vi "Manual Roller Control.vi"() -> (1 "Boolean":bool, 2 "Right Speed Out":dbl, 3 "Left Speed Out":dbl)   [LabVIEW 2014]
uses:
  Really Real Manual Align.ctl
  Robot Global Data.vi
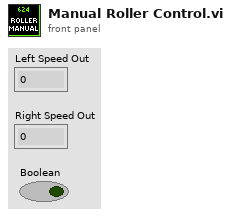
[diagram p1: front panel]
types:
  T1 = typedef "Really Real Manual Align.ctl" = enum16{"In", "Left", "Right", "Out", "Idle", "HP Load", "Speeds"}
  T2 = typedef "Dashboard Control Data.ctl" = cluster{"Cam Exposure":dbl, "Go to angle":dbl, "Steer PID Gains":cluster{"proportional gain (Kc)":dbl, "integral time (Ti, min)":dbl, "derivative time (Td, min)":dbl}, "Steer PID output Range":cluster{"output high":dbl, "output low":dbl}, "Pressure m \nValue":dbl, "Pressure b \nValue":dbl, "Roller Command Cluster ":T3, "Elevator":T4, "Encoder Control":T6, "Auton Settings":cluster{"Drive Dist Window Size":dbl}, "Drivetrain Settings":T7, "Lance":T8}
  T3 = typedef "Roller Control.ctl" = cluster{"Intake Speed":dbl, "Turn In Speed":dbl, "Unload Speed":dbl, "Turn Out Speed":dbl, "Ping Align Tolerance":dbl, "Tote Range Threshold":dbl, "Right Pot 0":dbl, "Pot Threshold":dbl, "Left Pot 0":dbl, "Manual 0s?":bool, "Right Pot Scale":dbl, "Left Pot Scale":dbl, "0 wait time":i32, "Zero Pots":bool, "Min Elevator Height":dbl, "Eject Time":dbl, "Eject US Threshold":dbl, "Anti-Twitch Time":u32, "Ping Caring Threshold":dbl, "Pot Diff Threshold":dbl, "Pinch Sustain":u32, "Absorb Give Up Threshold":dbl, "Untip In Threshold":dbl, "Untip Grab Range":dbl, "Ultrasonic Hold Time":u32, "Landscape Absorb Time":u32, "Pot Use Wait Time":u32, "Can Turn Stop Range":dbl, "Ignore Pressure":bool, "HP Load Speed":dbl}
  T4 = typedef "Elevator DB Control.ctl" = cluster{"PID Output Range":cluster{"output high":dbl, "output low":dbl}, "PID gains":cluster{"proportional gain (Kc)":dbl, "integral time (Ti, min)":dbl, "derivative time (Td, min)":dbl}, "Height Tolerance":sgl, " Encoder Constant":dbl, "Safe Mode Max Speed":sgl, "Eject Time":sgl, "Zeroing Speed":sgl, "Presets":T5, "Ping Detect Threshold":sgl, "Trashcan Detect Threshold":sgl, "Zero Filter Time":dbl, "Stabilizer Open Time":dbl, "Zero Creep Speed":dbl, "Max Current":dbl, "Current Trip Time":dbl, "Abort Pitch":dbl, "Finger m":dbl, "Finger b":dbl, "Finger max ":dbl, "Finger Stabilizer":dbl, "Finger Store":dbl, "Finger Stop Store":dbl, "Stabilizer Close Time":dbl, "HP Finger Store":dbl, "HP Finger Stop Store":dbl, "Finger min":dbl, "Unstick gain":dbl, "Roller Wait":dbl}
  T5 = typedef "Elevator Presets.ctl" = cluster{"Pickup 2 w/ Tote":sgl, "Pickup 2 w/ Trashcan":sgl, "Pickup 3 w/ Tote":sgl, "Pickup 3 w/ Trashcan":sgl, "Bottom":sgl, "Pickup 1 w/ Tote":sgl, "Pickup Trashcan":sgl, "Pickup 1 w/ Trashcan":sgl, "Eject":sgl, "Hold Low":sgl, "Step add height":sgl, "Untip Lift":dbl, "Drop Stack":dbl, "HP Load Hold":dbl, "HP Load Drop":dbl, "HP Load Finger":dbl, "HP Load Hold Can":dbl, "Store can max":dbl, "HP Drag Score":dbl, "HP Store can max":dbl, "HP Drag Finish":dbl, "HP Carry min":dbl, "HP Finger Anti-Crash":dbl, "Finger trashcan avoid":dbl}
  T6 = typedef "Encoder Control.ctl" = cluster{"Left Tick Constant":dbl, "Right Tick Constant":dbl, "Center Tick Constant":dbl, "Reset?":bool, "Y Dist":cluster{"PID gains":cluster{"proportional gain (Kc)":dbl, "integral time (Ti, min)":dbl, "derivative time (Td, min)":dbl}}, "X Dist":cluster{"PID gains":cluster{"proportional gain (Kc)":dbl, "integral time (Ti, min)":dbl, "derivative time (Td, min)":dbl}}, "Y Stop Thresh":dbl, "Y Stop Speed":dbl, "X Stop Thresh":dbl, "X Stop Speed":dbl}
  T7 = typedef "Drivetrain Settings.ctl" = cluster{"Gyro Tolerance":sgl, "Strafe Correct max steer":sgl, "Strafe Timer Wait":sgl, "Throttle Ramp (ms)":sgl, "Strafe Ramp (ms)":sgl, "Angular rate compensation":bool, "Throttle to Rate Scale":sgl, "Rate compensation gain":sgl, "Creep Steer":sgl, "Creep Throttle":sgl}
  T8 = typedef "Pike DB Controls.ctl" = cluster{"Down Speed":dbl, "Up Speed":dbl, "Max Down Time":dbl, "Max Up Time":dbl, "Current Limit":dbl}
  T9 = typedef "Roller Manual Bools.ctl" = cluster{"Manual Claw":bool, "Manual Align":T1, "Left Speed":dbl, "Right Speed":dbl}
  T10 = typedef "Roller Modes.ctl" = cluster{"Auto Roller Command":T11, "Roller Mode":T12, "Override Intake Speed":dbl}
  T11 = typedef "Auto Roller Commands.ctl" = enum16{"Drag Tote", "Grab Tote", "Idle", "Eject Tote", "Untip Can", "Grab Can"}
  T12 = typedef "Roller Mode Enum.ctl" = enum16{"Manual", "Safe", "Auto"}
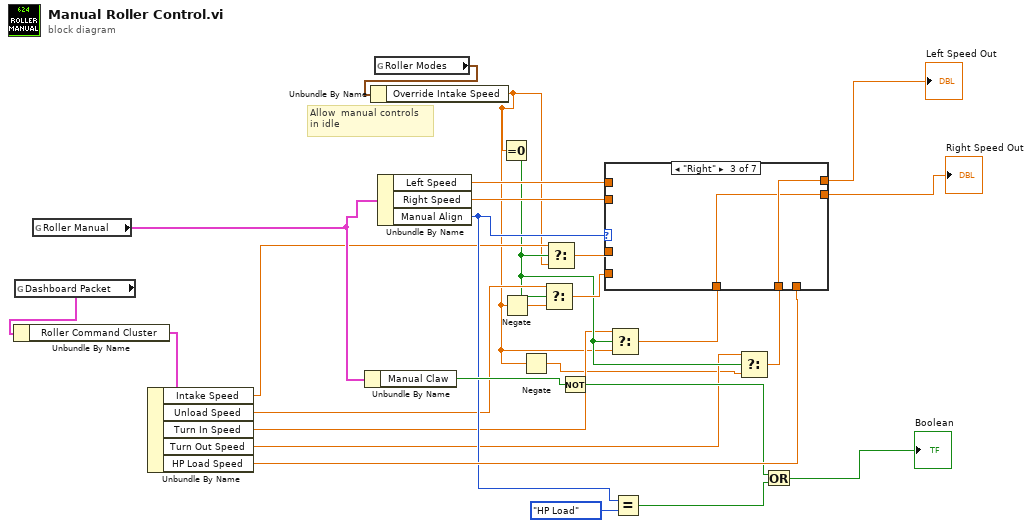
[diagram p0: block diagram]
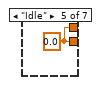
[diagram p5: hidden frame]
diagram:
  # "Allow  manual controls\nin idle"
  n1 = global read "Robot Global Data.vi" "Dashboard Packet"() -> (w24:T2)
  n2 = Unbundle By Name(w24) -> ("Roller Command Cluster"=w23:T3)
  n3 = global read "Robot Global Data.vi" "Roller Manual"() -> (w22:T9)
  n4 = Unbundle By Name(w23) -> ("Intake Speed"=w8:dbl, "Unload Speed"=w12:dbl, "Turn In Speed"=w5:dbl, "Turn Out Speed"=w4:dbl, "HP Load Speed"=w21:dbl)
  n5 = Unbundle By Name(w22) -> ("Manual Claw"=w27:bool)
  n6 = global read "Robot Global Data.vi" "Roller Modes"() -> (w13:T10)
  n7 = Unbundle By Name(w13) -> ("Override Intake Speed"=w1:dbl)
  n8 = Unbundle By Name(w22) -> ("Left Speed"=w15:dbl, "Right Speed"=w14:dbl, "Manual Align"=w19:T1)
  n9 = Equal To 0?(x=w1) -> (x = 0?=w7:bool)
  n10 = Negate(x=w1) -> (-x=w11:dbl)
  n11 = Negate(x=w1) -> (-x=w2:dbl)
  n12 = Select(t=w12, s=w7, f=w11) -> (s? t:f=w10:dbl)
  n13 = Select(t=w8, s=w7, f=w1) -> (s? t:f=w9:dbl)
  n14 = Not(x=w27) -> (.not. x?=w18:bool)
  n15 = Select(t=w5, s=w7, f=w1) -> (s? t:f=w6:dbl)
  n16 = Equal?(x=w19, y=Really_Real_Manual_Align."HP Load") -> (x = y?=w17:bool)
  n17 = Select(t=w4, s=w7, f=w2) -> (s? t:f=w3:dbl)
  n18 = case shown="\"Right\"" w19 {
    tunnel: [w28 w30 w31 w33 w34 w35 w36] -> w26
    tunnel: w9 -> [w28 _ _ _ _ _ _]
    tunnel: [w28 w29 w32 w33 w34 w35 w37] -> w25
    tunnel: w3 -> [_ w30 w32 _ _ _ _]
    tunnel: w21 -> [_ _ _ _ _ w35 _]
    tunnel: w15 -> [_ _ _ _ _ _ w37]
    tunnel: w14 -> [_ _ _ _ _ _ w36]
    tunnel: w10 -> [_ _ _ w33 _ _ _]
    tunnel: w6 -> [_ w29 w31 _ _ _ _]
    frame "In", Default {
    }
    frame "Left" {
    }
    frame "Right" {
    }
    frame "Out" {
    }
    frame "Idle" {
      w34 = 0.0 ("Unload Speed")
    }
    frame "HP Load" {
    }
    frame "Speeds" {
    }
  }
  "Right Speed Out" <- w26
  "Left Speed Out" <- w25
  n19 = Or(x=w18, y=w17) -> (x .or. y?=→"Boolean":bool)
